vi "DigUpPix.vi"(7 "Raw Data File":path, 9 "Result files to read":path[](array[path]), 11 "Cursor index":i32) -> ()   [LabVIEW 2022 SP3]
uses:
  Anemometry/Anemometry Sub Vis/Data_plotting_vis/Results_plotter_Global.vi
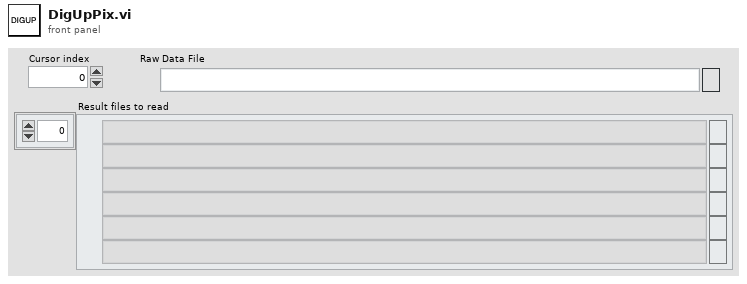
[diagram p1: front panel]
types:
  T1 = enum32{"Invalid", "Standard", "Closed", "Hidden", "Minimized", "Maximized"}
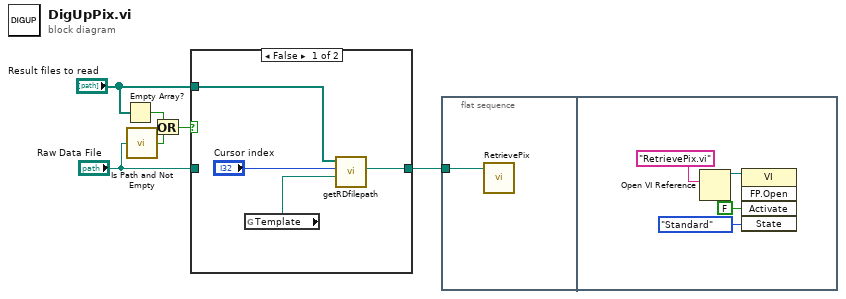
[diagram p0: block diagram]
diagram:
  n1 = Empty Array?(array="Result files to read") -> (empty?=w1:bool)
  n2 = call <vilib>:"Is Path and Not Empty.vi"("path"="Raw Data File") -> ("Is Path and Not Empty?"=w4:bool)  [unwired: 4 in]
  n3 = Or(x=w1, y=w4) -> (x .or. y?=w2:bool)
  n4 = case shown="False" w2 {
    tunnel: [w10 w11] -> w6
    tunnel: "Raw Data File" -> [_ w11]
    tunnel: "Result files to read" -> [w7 _]
    frame False {
      n5 = global read "Results_plotter_Global.vi" "Template"() -> (w8:path)
      n6 = call "getRDfilepath.vi"("templatePath"=w8, "rowIndex"="Cursor index", "Result files to read"=w7) -> ("rawDataPath"=w10:path)  [unwired: 6 in, 2 out]
    }
    frame True {
    }
  }
  n7 = flat-sequence {
    tunnel: w6 -> [w12]
    frame #0 {
      n8 = call "RetrievePix.vi"("RawDataFile"=w12) -> ()  [unwired: 8 in, 3 out]
    }
    frame #1 {
      n9 = Open VI Reference(vi path="RetrievePix.vi") -> (vi reference=w16:refnum<vi>)  [unwired: 5 in, 1 out]
      n10 = invoke class="VI" method="FP.Open"(reference=w16, "Activate"=FALSE ("Activate?"), "State"=T1."Standard") -> ()  [unwired: 2 in, 5 out]
    }
  }
